vi "AddNode__slk_msxml.vi"(0 "document in":refnum<class "msxml document.lvclass">, 5 "parent node in":refnum<class "msxml node.lvclass">, 7 "node name":string, 9 "text":string, 11 "error in (no error)":errorcluster, 12 "attributes":T1) -> (4 "document out":refnum<class "msxml document.lvclass">, 6 "new node out":refnum<class "msxml node.lvclass">, 15 "error out":errorcluster)   [LabVIEW 2020, in "MSXML.lvlib" / "msxml document.lvclass"]
doc: "Adds a branch to a MSXML Document."
uses:
  msxml document.lvclass
  Type Definition/Attributes__slk_msxml.ctl
  Type Definition/Attribute__slk_msxml.ctl
  MSXML Node/msxml node.lvclass
  msxml document.lvclass/msxml document.ctl
  MSXML.lvlib
panel:
  # "AddNode__slk_msxml.vi\n\nAdds a branch to a MSXML Document.\n\nNOTICE -- YOU MUST LEAVE THIS NOTICE IN PLACE.\n\nCopyright (c) 2004-2010 Shawn Liu <shawn.liu.cn@gmail.com>\n\nAll rights reserved."
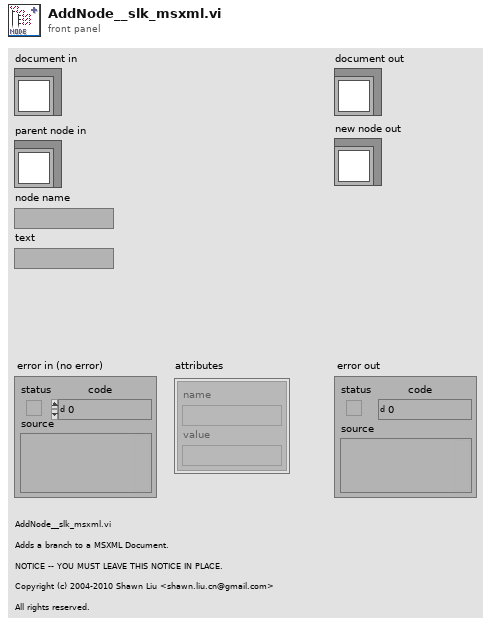
[diagram p1: front panel]
types:
  T1 = typedef "MSXML.lvlib/Attributes__slk_msxml.ctl" = T2[]
  T2 = typedef "MSXML.lvlib/Attribute__slk_msxml.ctl" = cluster{"name":string, "value":string}
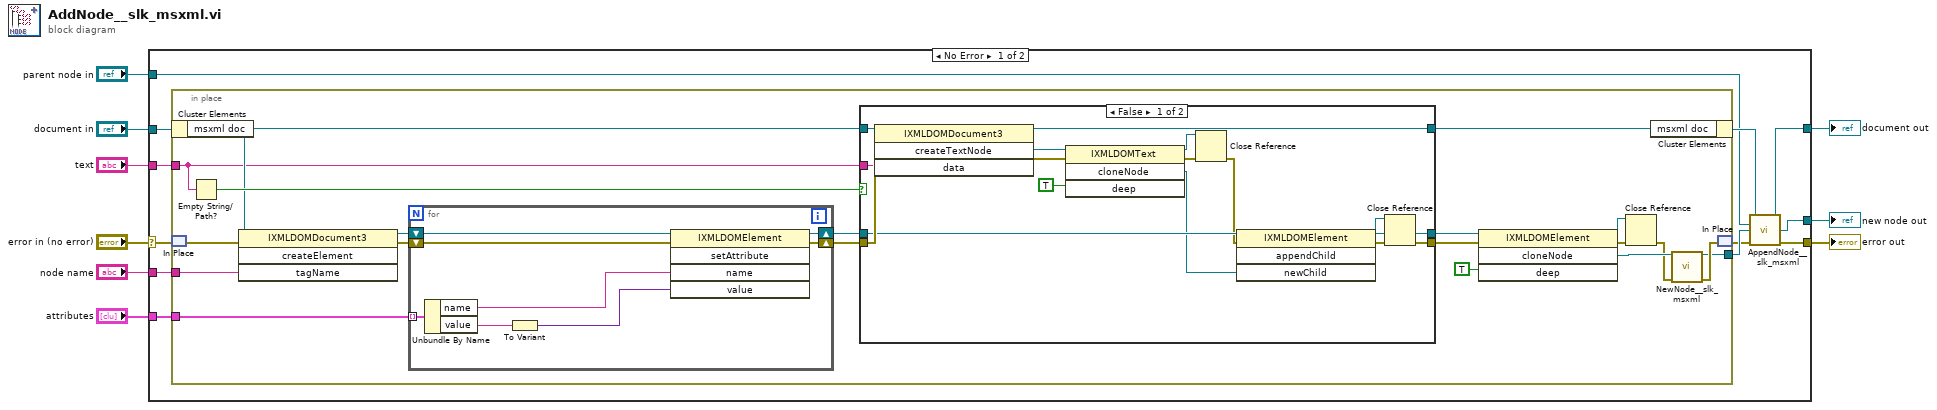
[diagram p0: block diagram]
diagram:
  n1 = case shown="No Error" "error in (no error)" {
    selector: "error in (no error)" -> [w18 w70]
    tunnel: "node name" -> [w21 _]
    tunnel: [w17 w70] -> w8
    tunnel: "attributes" -> [w20 _]
    tunnel: "document in" -> [w19 w69]
    tunnel: [w15 w69] -> w4
    tunnel: "parent node in" -> [w14 _]
    tunnel: [w11 _] -> w2
    tunnel: "text" -> [w10 _]
    frame No Error {
      n2 = in-place {
        in-place-border: w21 -> [w41]
        in-place-border: w20 -> [w35]
        in-place-border: [w30] -> w13
        in-place-border: w10 -> [w22]
        n3 = in-place-cluster #1(w19) -> ("msxml doc"=w28:refnum<k7>)
        n4 = in-place-match #2(w18) -> (w34:errorcluster)
        n5 = Empty String/Path?(string/path=w22) -> (empty?=w29:bool)
        n6 = invoke class="IXMLDOMDocument3" method="createElement"(reference=w28, error in=w34, "tagName"=w41) -> (error out=w39:errorcluster, "createElement"=w40:refnum<k7>)  [unwired: 1 in, 2 out]
        n7 = for {
          shift-right: [w66] -> w27
          shift-left: w39 -> [w62]
          shift-right: [w67] -> w26
          shift-left: w40 -> [w68]
          tunnel: w35 -> [w63] mode=indexing
          n8 = Unbundle By Name(w63) -> ("name"=w64:string, "value"=w65:string)
          n9 = To Variant(anything=w65) -> (Variant=w61:variant)
          n10 = invoke class="IXMLDOMElement" method="setAttribute"(reference=w68, error in=w62, "name"=w64, "value"=w61) -> (reference out=w67:refnum<k7>, error out=w66:errorcluster)  [unwired: 1 in, 3 out]
        }
        n11 = case shown="False" w29 {
          tunnel: w28 -> [w54 w59]
          tunnel: w27 -> [w53 w58]
          tunnel: w26 -> [w50 w60]
          tunnel: [w47 w60] -> w25
          tunnel: [w46 w59] -> w24
          tunnel: [w44 w58] -> w23
          tunnel: w22 -> [w42 _]
          frame False {
            n12 = invoke class="IXMLDOMDocument3" method="createTextNode"(reference=w54, error in=w53, "data"=w42) -> (reference out=w46:refnum<k7>, error out=w56:errorcluster, "createTextNode"=w55:refnum<k7>)  [unwired: 1 in, 1 out]
            n13 = invoke class="IXMLDOMText" method="cloneNode"(reference=w55, error in=w56, "deep"=TRUE) -> (reference out=w51:refnum<k7>, error out=w52:errorcluster, "cloneNode"=w48:refnum<k7>)  [unwired: 1 in, 1 out]
            n14 = Close Reference(reference=w51, error in (no error)=w52) -> (error out=w49:errorcluster)
            n15 = invoke class="IXMLDOMElement" method="appendChild"(reference=w50, error in=w49, "newChild"=w48) -> (reference out=w47:refnum<k7>, error out=w45:errorcluster, "appendChild"=w43:refnum<k7>)  [unwired: 1 in, 1 out]
            n16 = Close Reference(reference=w43, error in (no error)=w45) -> (error out=w44:errorcluster)
          }
          frame True {
          }
        }
        n17 = invoke class="IXMLDOMElement" method="cloneNode"(reference=w25, error in=w23, "deep"=TRUE) -> (reference out=w36:refnum<k7>, error out=w37:errorcluster, "cloneNode"=w32:refnum<k7>)  [unwired: 1 in, 1 out]
        n18 = Close Reference(reference=w36, error in (no error)=w37) -> (error out=w31:errorcluster)
        n19 = in-place-cluster #1("msxml doc"=w24) -> (w16:refnum<class "msxml document.lvclass">)
        n20 = call "NewNode__slk_msxml.vi"("msxml node"=w32, "error in (no error)"=w31) -> ("node out"=w30:refnum<class "msxml node.lvclass">, "error out"=w33:errorcluster)  [unwired: 12 in]
        n21 = in-place-match #2(w33) -> (w12:errorcluster)
      }
      n22 = call "AppendNode__slk_msxml.vi"("document in"=w16, "parent node in"=w14, "new node in"=w13, "error in (no error)"=w12) -> ("document out"=w15:refnum<class "msxml document.lvclass">, "new node out"=w11:refnum<class "msxml node.lvclass">, "error out"=w17:errorcluster)  [unwired: 8 in, 1 out]
    }
    frame Error {
    }
  }
  "document out" <- w4
  "error out" <- w8
  "new node out" <- w2
